vi "receiveFromFPGA.vi"(8 "error in (no error)":errorcluster, 11 "ModbusPort1 in":refnum<class "ModbusPort3.lvclass">) -> (0 "error out":errorcluster, 2 "Data":u16[](array[numeric]), 3 "ModbusPort1 out":refnum<class "ModbusPort3.lvclass">)   [LabVIEW 2015, in "ModbusPort3.lvclass"]
uses:
  ModbusPort3.lvclass
  Modbus/Modbus.lvclass/Modbus.ctl
  <vilib>/Utility/error.llb/Error Cluster From Error Code.vi
  <vilib>/rvi/errors/niLvFpgaAdjustHostInterfaceError.vi
  <vilib>/rvi/interface/nirviMethod/nirviMethod.xnode
  Modbus/Modbus.lvclass
  <vilib>/FPGAPlugInAG/Dynamic/niLvFpga_ReadFifo_Dynamic.vi
  <vilib>/rvi/errors/niLvFpgaMergeErrorWithErrorCode.vi
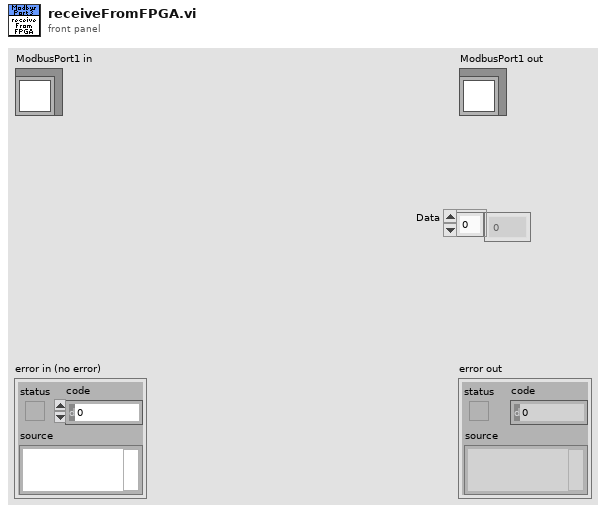
[diagram p1: front panel]
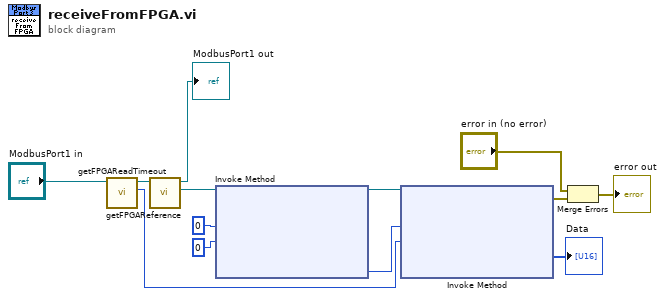
[diagram p0: block diagram]
diagram:
  n1 = call "getFPGAReadTimeout.vi"("Modbus in"="ModbusPort1 in") -> ("FPGAReadTimeout"=w7:i32, "Modbus out"=w12:refnum<class "ModbusPort3.lvclass">)  [unwired: 9 in]
  n2 = call "getFPGAReference.vi"("Modbus in"=w12) -> ("FPGAReference"=w11:refnum<k20>, "Modbus out"=→"ModbusPort1 out":refnum<class "ModbusPort3.lvclass">)  [unwired: 9 in]
  n3 = xnode "Invoke Method"("FPGA VI Reference In"=w11, "Number of Elements"=u32 0, "Timeout (ms)"=0) -> ("FPGA VI Reference Out"=w6:refnum<k20>, "Elements Remaining"=w8:u32)  [unwired: 1 in, 2 out]
  n4 = xnode "Invoke Method"("FPGA VI Reference In"=w6, "Number of Elements"=w8, "Timeout (ms)"=w7) -> ("error out"=w3:errorcluster, "Data"=→"Data":u16[])  [unwired: 1 in, 2 out]
  n5 = Merge Errors("error in (no error)", w3) -> (→"error out":errorcluster)
